vi "ProgressBar Window.vi"(8 "error in (no error)":errorcluster, 11 "Progress bar window values input cluster":T1) -> (0 "error out":errorcluster)   [LabVIEW 2020]
uses:
  Progress bar window values input cluster.ctl
  System.Windows.Forms
  <vilib>/Utility/miscctls.llb/LVPointTypeDef.ctl
  Global Variables/General Globals.vi
panel:
  in  "Acq ProgressBar":refnum<k24>(container)
  out "Acquisition message":string
  in  "Logging ProgressBar":refnum<k24>(container)
  out "Overall Progress":u8(slide) max=1 step=1 scale=0.0..100.0
  out "Message":string
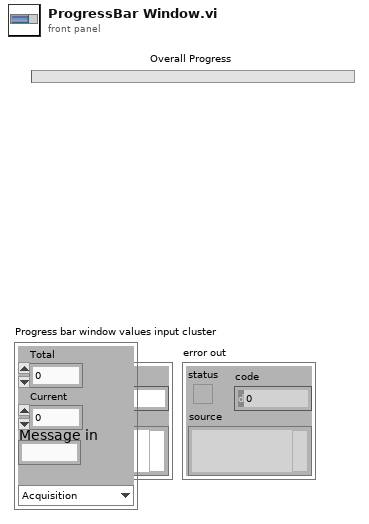
[diagram p1: front panel]
types:
  T1 = typedef "Progress bar window values input cluster.ctl" = cluster{"Total":i32, "Current":i32, "Message in":string, "Sender":enum16{"Acquisition", "Logging", "File gen"}}
  T2 = typedef "LVPointTypeDef.ctl" = cluster{"Horizontal":i16, "Vertical":i16}
  T3 = enum8{"Enabled", "Disabled", "Disabled and Grayed Out"}
  T4 = typedef "Progressbar window queue ref.ctl" = refnum<queue>
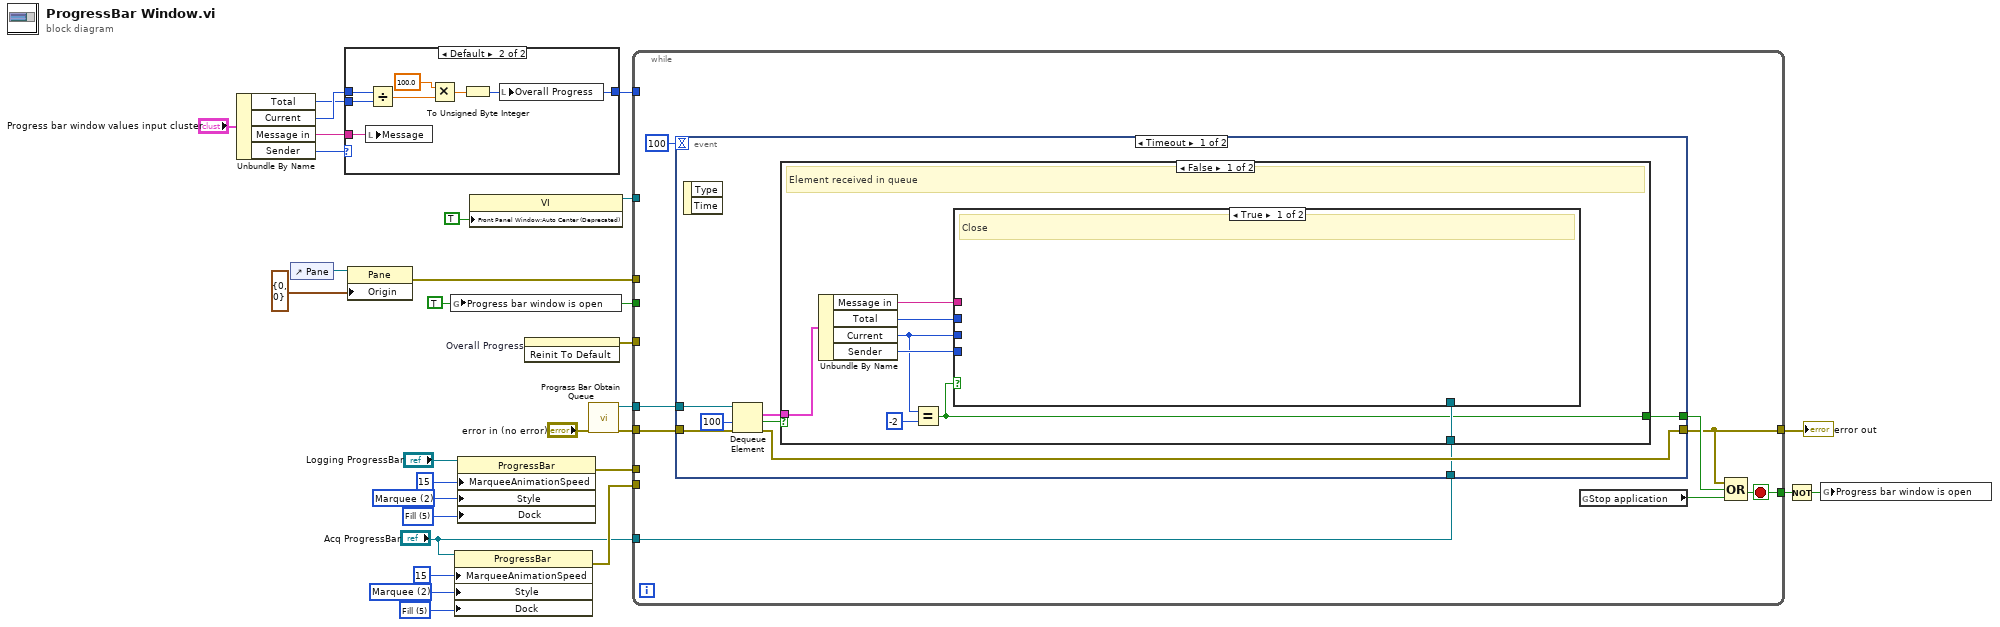
[diagram p0: block diagram]
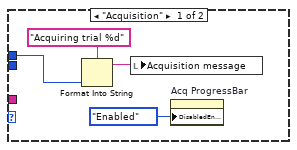
[diagram p2: hidden frame]
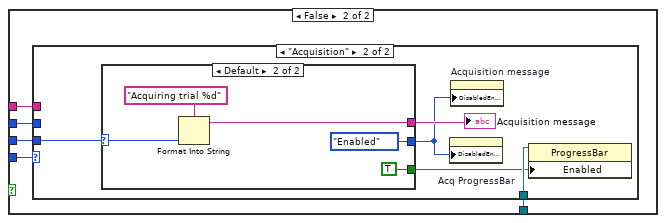
[diagram p3: hidden frame]
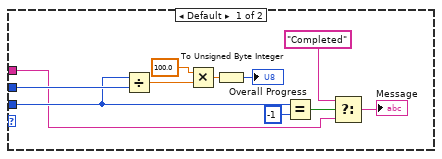
[diagram p4: hidden frame]
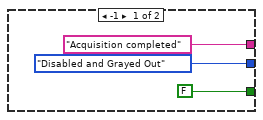
[diagram p5: hidden frame]
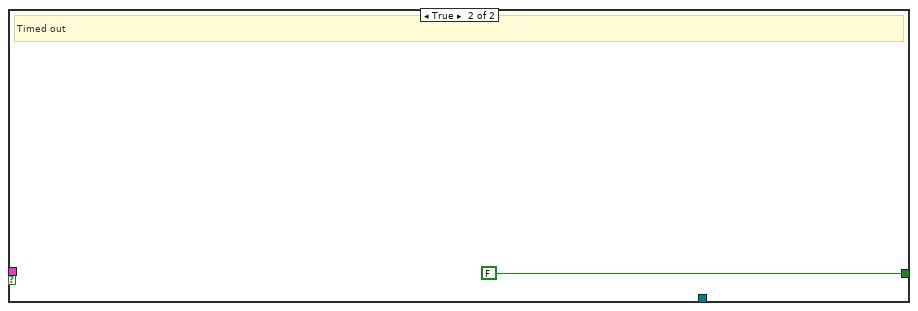
[diagram p6: hidden frame]
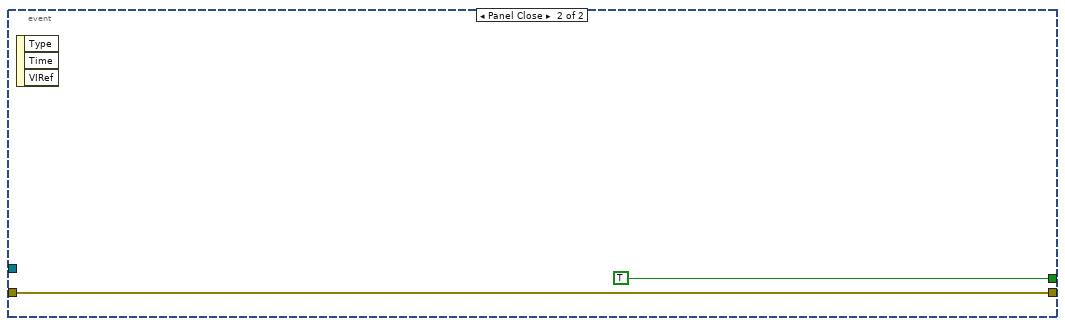
[diagram p7: hidden frame]
diagram:
  w6 = 5 items=["None", "Top", "Bottom", "Left", "Right", "Fill"] ("Dock")
  w4 = 2 items=["Blocks", "Continuous", "Marquee"] ("Style")
  w12 = 5 items=["None", "Top", "Bottom", "Left", "Right", "Fill"] ("Dock")
  w15 = 2 items=["Blocks", "Continuous", "Marquee"] ("Style")
  w26 = TRUE ("Progress bar window is open")
  n1 = Unbundle By Name("Progress bar window values input cluster") -> ("Total"=w22:i32, "Current"=w23:i32, "Message in"=w16:string, "Sender"=w7:enum16{"Acquisition", "Logging", "File gen"})
  n2 = control-ref of="Pane"() -> (w10:refnum<vi>)
  n3 = case shown="Default" w7 {
    tunnel: w23 -> [w32 w37]
    tunnel: w22 -> [_ w36]
    tunnel: [_ w35] -> w21
    tunnel: w16 -> [_ w34]
    frame "Acquisition" {
      n4 = Format Into String(format string="Acquiring trial %d", w32) -> (resulting string=w31:string)  [unwired: 2 in, 1 out]
      n5 = local write "Acquisition message"(w31) -> ()
      n6 = property on="Acq ProgressBar" class="AXCont"("DisabledEnum"=T3."Enabled" ("Disabled")) -> ()  [unwired: 2 in, 2 out]
    }
    frame Default {
      n7 = local write "Message"(w34) -> ()
      n8 = Divide(x=w37, y=w36) -> (x/y=w40:dbl)
      n9 = Multiply(x=100.0, y=w40) -> (x*y=w38:dbl)
      n10 = To Unsigned Byte Integer(number=w38) -> (unsigned 8bit integer=w35:u8)
      n11 = local write "Overall Progress"(w35) -> ()
    }
  }
  n12 = property class="Pane"(reference=w10, "Origin"=T2 {"Horizontal"=0, "Vertical"=0}) -> (error out=w8:errorcluster)  [unwired: 1 in, 1 out]
  n13 = global write "General Globals.vi" "Progress bar window is open"(w26) -> ()
  n14 = property class="ProgressBar"(reference="Acq ProgressBar", "MarqueeAnimationSpeed"=15, "Style"=w4, "Dock"=w6) -> (error out=w3:errorcluster)  [unwired: 1 in, 1 out]
  n15 = property class="ProgressBar"(reference="Logging ProgressBar", "MarqueeAnimationSpeed"=15, "Style"=w15, "Dock"=w12) -> (error out=w11:errorcluster)  [unwired: 1 in, 1 out]
  n16 = property on="Property Node" class="VI"("Front Panel Window:Auto Center (Deprecated)"=TRUE ("Front Panel Window:Auto Center")) -> (reference out=w27:refnum<vi>)  [unwired: 2 in, 1 out]
  n17 = invoke on="Overall Progress" class="Slide (strict)" method="Reinit To Default"() -> (error out=w29:errorcluster)  [unwired: 3 in, 2 out]
  n18 = call "Prograss Bar Obtain Queue.vi"("error in"="error in (no error)") -> ("error out"=w19:errorcluster, "Progressbar window queue ref"=w20:T4)  [unwired: 9 in]
  n19 = while {
    tunnel: w29 -> [_]
    tunnel: w27 -> [_]
    tunnel: w26 -> [_]
    tunnel: [w46] -> w25
    tunnel: w21 -> [_]
    tunnel: w20 -> [w45]
    tunnel: w19 -> [w44]
    tunnel: [w43] -> w17
    tunnel: w11 -> [_]
    tunnel: w8 -> [_]
    tunnel: w3 -> [_]
    tunnel: "Acq ProgressBar" -> [w42]
    stop <- w46 stop-if-true
    n20 = event shown="[0] Timeout" {
      selector: _ -> [_ _]
      dyn-events: _ -> [_ _]
      timeout: 100 -> [_ _]
      tunnel: [w53 TRUE] -> w48
      tunnel: w45 -> [w52 _]
      tunnel: w44 -> [w51 w95]
      tunnel: [w50 w95] -> w43
      tunnel: w42 -> [w49 _]
      event Timeout {
        n21 = event-data() -> ()  [unwired: 1 in, 2 out]
        n22 = Dequeue Element(queue=w52, timeout in ms (-1)=100, error in (no error)=w51) -> (element=w55:T1, timed out?=w54:bool, error out=w50:errorcluster)  [unwired: 1 out]
        n23 = case shown="False" w54 {
          tunnel: w55 -> [w63 _]
          tunnel: [w57 FALSE] -> w53
          tunnel: w49 -> [w60 _]
          frame False {
            # "Element received in queue"
            n24 = Unbundle By Name(w63) -> ("Message in"=w62:string, "Total"=w64:i32, "Current"=w59:i32, "Sender"=w61:enum16{"Acquisition", "Logging", "File gen"})
            n25 = Equal?(x=w59, y=-2) -> (x = y?=w57:bool)
            n26 = case shown="True" w57 {
              tunnel: w64 -> [_ w69]
              tunnel: w62 -> [_ w68]
              tunnel: w61 -> [_ w67]
              tunnel: w60 -> [_ w66]
              tunnel: w59 -> [_ w65]
              frame True {
                # "Close"
              }
              frame False {
                n27 = case shown="\"Acquisition\"" w67 {
                  tunnel: w69 -> [w80 _]
                  tunnel: w65 -> [w75 w85]
                  tunnel: w68 -> [w71 _]
                  tunnel: w66 -> [_ w82]
                  frame Default {
                    n28 = Divide(x=w75, y=w80) -> (x/y=w77:dbl)
                    n29 = Multiply(x=100.0, y=w77) -> (x*y=w79:dbl)
                    n30 = To Unsigned Byte Integer(number=w79) -> (unsigned 8bit integer=→"Overall Progress":u8)
                    n31 = Equal?(x=w75, y=-1) -> (x = y?=w73:bool)
                    n32 = Select(t="Completed", s=w73, f=w71) -> (s? t:f=→"Message":string)
                  }
                  frame "Acquisition" {
                    n33 = case shown="Default" w85 {
                      selector: w85 -> [_ w92]
                      tunnel: ["Acquisition completed" w91] -> w84
                      tunnel: [T3."Disabled and Grayed Out" ("Disabled") T3."Enabled" ("Disabled")] -> w83
                      tunnel: [FALSE ("Enabled") TRUE ("Enabled")] -> w81
                      frame -1 {
                      }
                      frame Default {
                        n34 = Format Into String(format string="Acquiring trial %d", w92) -> (resulting string=w91:string)  [unwired: 2 in, 1 out]
                      }
                    }
                    "Acquisition message" <- w84
                    n35 = property on="Acq ProgressBar" class="AXCont"("DisabledEnum"=w83) -> ()  [unwired: 2 in, 2 out]
                    n36 = property on="Acquisition message" class="Str"("DisabledEnum"=w83) -> ()  [unwired: 2 in, 2 out]
                    n37 = property class="ProgressBar"(reference=w82, "Enabled"=w81) -> ()  [unwired: 1 in, 2 out]
                  }
                }
              }
            }
          }
          frame True {
            # "Timed out"
          }
        }
      }
      event Panel Close {
        n38 = event-data() -> ()  [unwired: 1 in, 3 out]
      }
    }
    n39 = global read "General Globals.vi" "Stop application"() -> (w41:bool)
    n40 = Compound Arithmetic op=OR(w43, w48, w41) -> (w46:bool)
  }
  "error out" <- w17
  n41 = Not(x=w25) -> (.not. x?=w1:bool)
  n42 = global write "General Globals.vi" "Progress bar window is open"(w1) -> ()
